vi "ubinary_load.vi"(8 "error in":errorcluster, 9 "control":string, 10 "file (use dialog)":path, 11 "VI":refnum<vi>) -> (0 "error out":errorcluster)   [LabVIEW 2012]
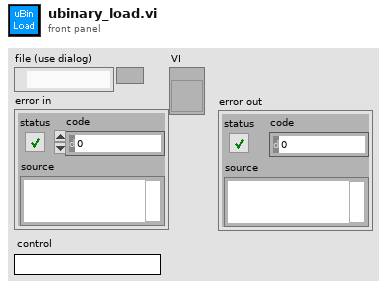
[diagram p1: front panel]
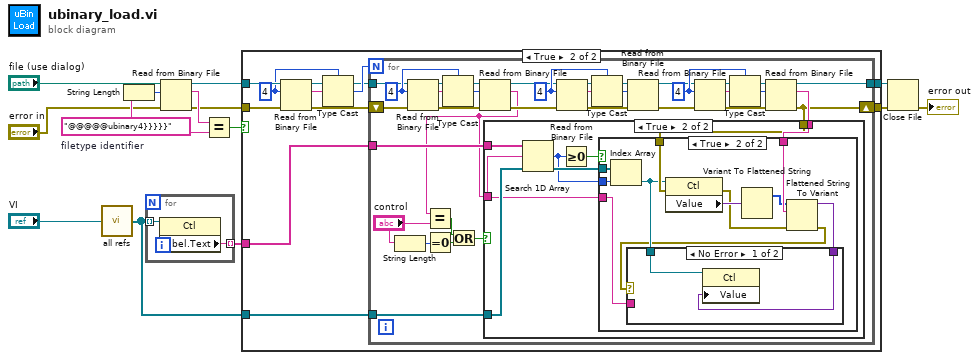
[diagram p0: block diagram]
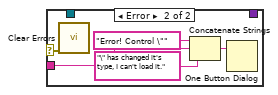
[diagram p5: hidden frame]
diagram:
  w12 = "@@@@@ubinary4}}}}}"  # filetype identifier
  n1 = call "all refs.vi"("VI"="VI") -> ("all controls"=w1:refnum<vi>[])
  n2 = String Length(string=w12) -> (length=w13:i32)
  n3 = for {
    tunnel: w1 -> [w16] mode=indexing
    tunnel: [w15] -> w7 mode=indexing
    n4 = property class="Ctl"(reference=w16) -> ("Label.Text"=w15:string)  [unwired: 1 in, 2 out]
  }
  n5 = Read from Binary File(8:"error in", 10:w13, 11:"file (use dialog)") -> (0:w8:errorcluster, 2:w11:string, 3:w10:refnum<file>)  [unwired: 3 in, 1 out]
  n6 = Equal?(x=w11, y=w12) -> (x = y?=w9:bool)
  n7 = case shown="True" w9 {
    tunnel: [w18 w19] -> w14
    tunnel: w10 -> [w18 w29]
    tunnel: w8 -> [w17 w24]
    tunnel: w7 -> [_ w23]
    tunnel: [w17 w22] -> w6
    tunnel: w1 -> [_ w21]
    frame False {
    }
    frame True {
      w27 = 4 ("count (1)")
      n8 = Read from Binary File(8:w24, 10:w27, 11:w29) -> (0:w25:errorcluster, 2:w28:string, 3:w20:refnum<file>)  [unwired: 3 in, 1 out]
      n9 = Type Cast(type=w27, x=w28) -> (*(type *) &x=w26:i32)
      n10 = for {
        N: w26 -> [_]
        tunnel: w20 -> [w59]
        shift-right: [w36] -> w22
        shift-left: w25 -> [w55]
        tunnel: w23 -> [w54]
        tunnel: w21 -> [w39]
        tunnel: [w37] -> w19
        w48 = 4 ("count (1)")
        w49 = 4 ("count (1)")
        w61 = 4 ("count (1)")
        n11 = String Length(string="control") -> (length=w32:i32)
        n12 = Read from Binary File(8:w55, 10:w61, 11:w59) -> (0:w56:errorcluster, 2:w60:string, 3:w58:refnum<file>)  [unwired: 3 in, 1 out]
        n13 = Equal To 0?(x=w32) -> (x = 0?=w31:bool)
        n14 = Type Cast(type=w61, x=w60) -> (*(type *) &x=w57:i32)
        n15 = Read from Binary File(8:w56, 10:w57, 11:w58) -> (0:w42:errorcluster, 2:w35:string, 3:w43:refnum<file>)  [unwired: 3 in, 1 out]
        n16 = Equal?(x=w35, y="control") -> (x = y?=w33:bool)
        n17 = Or(x=w33, y=w31) -> (x .or. y?=w34:bool)
        n18 = Read from Binary File(8:w42, 10:w49, 11:w43) -> (0:w53:errorcluster, 2:w50:string, 3:w51:refnum<file>)  [unwired: 3 in, 1 out]
        n19 = Type Cast(type=w49, x=w50) -> (*(type *) &x=w52:i32)
        n20 = Read from Binary File(8:w53, 10:w52, 11:w51) -> (0:w41:errorcluster, 3:w40:refnum<file>)  [unwired: 3 in, 2 out]
        n21 = Read from Binary File(8:w41, 10:w48, 11:w40) -> (0:w44:errorcluster, 2:w47:string, 3:w46:refnum<file>)  [unwired: 3 in, 1 out]
        n22 = Type Cast(type=w48, x=w47) -> (*(type *) &x=w45:i32)
        n23 = Read from Binary File(8:w44, 10:w45, 11:w46) -> (0:w36:errorcluster, 2:w38:string, 3:w37:refnum<file>)  [unwired: 3 in, 1 out]
        n24 = case shown="True" w34 {
          tunnel: w54 -> [_ w68]
          tunnel: w39 -> [_ w66]
          tunnel: w38 -> [_ w64]
          tunnel: w35 -> [_ w63]
          tunnel: w36 -> [_ w62]
          frame False {
          }
          frame True {
            n25 = Search 1D Array(1D array=w68, element=w63) -> (index of element=w65:i32)  [unwired: 1 in]
            n26 = Greater Or Equal To 0?(x=w65) -> (x >= 0?=w67:bool)
            n27 = case shown="True" w67 {
              tunnel: w66 -> [_ w79]
              tunnel: w65 -> [_ w78]
              tunnel: w64 -> [_ w77]
              tunnel: w63 -> [_ w69]
              tunnel: w62 -> [_ w73]
              frame False {
              }
              frame True {
                n28 = Index Array(array=w79, index=w78) -> (element=w72:refnum<vi>)
                n29 = property class="Ctl"(reference=w72, error in=w73) -> (error out=w74:errorcluster, "Value"=w76:variant)  [unwired: 1 out]
                n30 = Variant To Flattened String(Variant=w76) -> (1:w75:i16[])  [unwired: 1 out]
                n31 = Flattened String To Variant(4:w74, 6:w77, 7:w75) -> (0:w71:errorcluster, 3:w70:variant)
                n32 = case shown="No Error" w71 {
                  selector: w71 -> [_ w86]
                  tunnel: w72 -> [w81 _]
                  tunnel: w70 -> [w80 _]
                  tunnel: w69 -> [_ w84]
                  frame No Error {
                    n33 = property class="Ctl"(reference=w81, "Value"=w80) -> ()  [unwired: 1 in, 2 out]
                  }
                  frame Error {
                    n34 = call <vilib>:"Clear Errors.vi"("error in (no error)"=w86) -> ()  [unwired: 6 in, 1 out]
                    n35 = Concatenate Strings("Error! Control \"" ("string"), w84, "\" has changed it's type, I can't load it." ("string")) -> (w85:string)
                    n36 = One Button Dialog(message=w85) -> ()  [unwired: 1 in, 1 out]
                  }
                }
              }
            }
          }
        }
      }
    }
  }
  n37 = Close File(refnum=w14, error in=w6) -> (error out=→"error out":errorcluster)  [unwired: 1 out]
